vi "Commit Properties.vi"(8 "error in (no error)":errorcluster, 10 "resources":string, 11 "SLSC Remote in":refnum<class "SLSC Remote.lvclass">) -> (0 "error out":errorcluster, 3 "SLSC Remote out":refnum<class "SLSC Remote.lvclass">)   [LabVIEW 2015, in "SLSC Remote.lvclass"]
uses:
  SLSC Remote.lvclass
  <vilib>/NI/i3 JSON/JSON Generation/Create Value Files/Create Value - Object.vi
  <vilib>/NI/i3 JSON/JSON Generation/Add Object Parameter Files/Add Object Parameter - String.vi
  <vilib>/NI/NI JSONRPC Server Framework/Classes/Server/Format Client Request (Auto-Increment).vi
  <vilib>/httpClient/POSTBuffer.vi
  <vilib>/NI/NI JSONRPC Server Framework/Classes/Server/JSONRPC Server.lvclass
  <vilib>/NI/i3 JSON/i3-json.lvlib
  <vilib>/httpClient/LabVIEWHTTPClient.lvlib
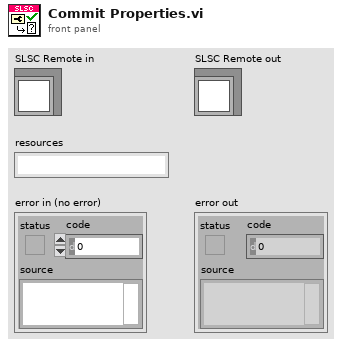
[diagram p1: front panel]
types:
  T1 = typedef "LabVIEWHTTPClient.lvlib/ClientHandle.ctl" = refnum<k1>
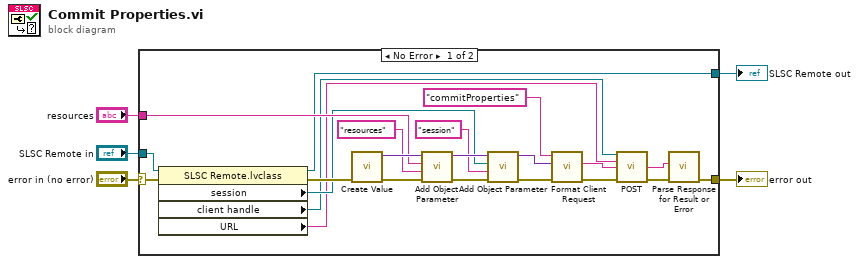
[diagram p0: block diagram]
diagram:
  n1 = case shown="No Error" "error in (no error)" {
    selector: "error in (no error)" -> [w22 w28]
    tunnel: "resources" -> [w26 _]
    tunnel: "SLSC Remote in" -> [w24 w29]
    tunnel: [w23 w29] -> w2
    tunnel: [w6 w28] -> w1
    frame No Error {
      n2 = property class="SLSC Remote.lvclass"(reference=w24, error in=w22) -> (reference out=w23:refnum<class "SLSC Remote.lvclass">, error out=w21:errorcluster, "session"=w15:refnum<k21>, "client handle"=w11:T1, "URL"=w10:string)
      n3 = call-poly <vilib>:"Create Value.vi"("error in (no error)"=w21) -> ("error out"=w20:errorcluster, "JSON Tree"=w27:variant)  [unwired: 9 in]
      n4 = call-poly <vilib>:"Add Object Parameter.vi"("error in (no error)"=w20, "Name"="resources", "String"=w26, "JSON Tree in (JSON Object)"=w27) -> ("error out"=w19:errorcluster, "JSON Tree out (JSON Object)"=w16:variant)  [unwired: 6 in]
      n5 = call-poly <vilib>:"Add Object Parameter.vi"("error in (no error)"=w19, "Name"="session", "String"=w15, "JSON Tree in (JSON Object)"=w16) -> ("error out"=w12:errorcluster, "JSON Tree out (JSON Object)"=w13:variant)  [unwired: 6 in]
      n6 = call-poly <vilib>:"Format Client Request.vi"("error in (no error)"=w12, "params"=w13, "method"="commitProperties") -> ("error out"=w9:errorcluster, "Request String"=w17:string)  [unwired: 7 in]
      n7 = call-poly <vilib>:"POST.vi"("client handle"=w11, "url"=w10, "buffer"=w17, "error in (no error)"=w9) -> ("body"=w8:string, "error out"=w7:errorcluster)  [unwired: 8 in, 2 out]
      n8 = call <vilib>:"Parse Response for Result or Error.vi"("error in"=w7, "Response String In"=w8) -> ("error out"=w6:errorcluster)  [unwired: 7 in, 2 out]
    }
    frame Error {
    }
  }
  "error out" <- w1
  "SLSC Remote out" <- w2
